vi "Equality within Range.vi"(1 "Range":dbl, 2 "Y":dbl, 3 "X":dbl) -> (0 "X = Y within Range?":bool)   [LabVIEW 2014]
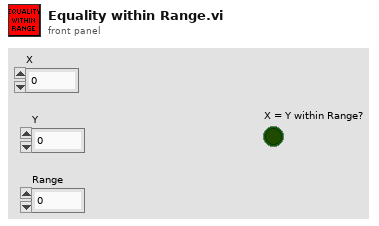
[diagram p1: front panel]
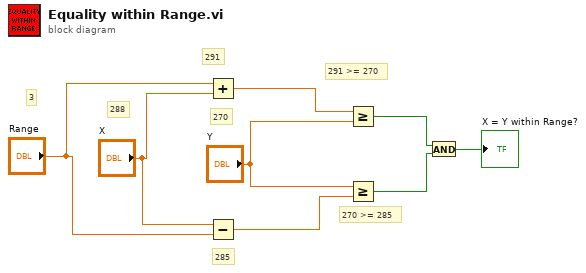
[diagram p0: block diagram]
diagram:
  # "291 >= 270"
  # "270 >= 285"
  # "285"
  # "291"
  # "270"
  # "3"
  # "288"
  n1 = Add(x="Range", y="X") -> (x+y=w4:dbl)
  n2 = Subtract(x="X", y="Range") -> (x-y=w6:dbl)
  n3 = Greater Or Equal?(x=w4, y="Y") -> (x >= y?=w3:bool)
  n4 = Greater Or Equal?(x="Y", y=w6) -> (x >= y?=w2:bool)
  n5 = And(x=w3, y=w2) -> (x .and. y?=→"X = Y within Range?":bool)
